vi "start_stage_trackball.vi"(2 "Enum":T1(ring), 3 "error in (no error)":errorcluster, 4 "Stage Controller port":refnum<visa-resource-name>="COM5") -> (0 "error out":errorcluster, 1 "Stage Controller port Out":refnum<visa-resource-name>="COM5")   [LabVIEW 2014]
uses:
  <vilib>/Instr/_visa.llb/VISA Configure Serial Port (Instr).vi
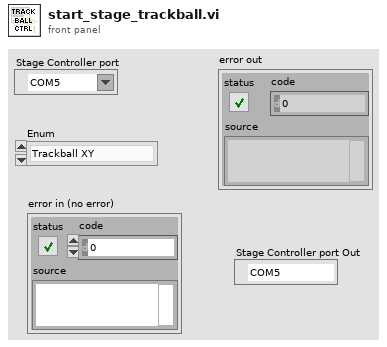
[diagram p1: front panel]
types:
  T1 = enum16{"Trackball XY", "Trackball Z", "Trackball OFF", ""}
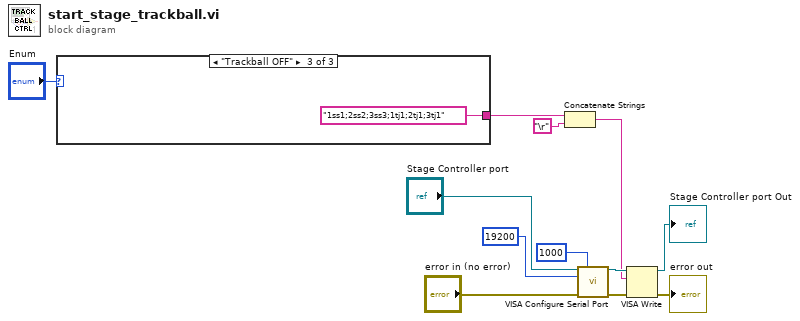
[diagram p0: block diagram]
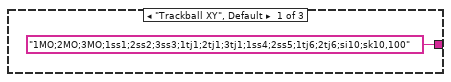
[diagram p2: hidden frame]
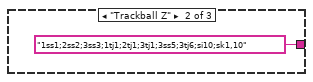
[diagram p3: hidden frame]
diagram:
  n1 = case shown="\"Trackball OFF\"" "Enum" {
    tunnel: ["1MO;2MO;3MO;1ss1;2ss2;3ss3;1tj1;2tj1;3tj1;1ss4;2ss5;1tj6;2tj6;si10;sk10,100" "1ss1;2ss2;3ss3;1tj1;2tj1;3tj1;3ss5;3tj6;si10;sk1,10" "1ss1;2ss2;3ss3;1tj1;2tj1;3tj1"] -> w7
    frame "Trackball XY", Default {
    }
    frame "Trackball Z" {
    }
    frame "Trackball OFF" {
    }
  }
  n2 = Concatenate Strings(w7, "\r") -> (w5:string)
  n3 = call-poly "VISA Configure Serial Port"("VISA resource name"="Stage Controller port", "timeout (10sec)"=u32 1000, "baud rate (9600)"=u32 19200, "error in (no error)"="error in (no error)") -> ("VISA resource name out"=w8:refnum<visa-resource-name>, "error out"=w4:errorcluster)  [unwired: 3 in, 7 out]
  n4 = VISA Write(VISA resource name=w8, write buffer=w5, error in (no error)=w4) -> (VISA resource name out=→"Stage Controller port Out":refnum<visa-resource-name>, error out=→"error out":errorcluster)  [unwired: 1 out]
